vi "Init.vi"(6 "dT (Auto)":dbl, 7 "Output Range":T1={"Min"=-50.0, "Max"=50.0}, 8 "error in (no error)":errorcluster, 11 "Parameters":T2={"P Band"=10.0, "I Gain"=0.5, "D Gain"=0.1, "F Gain"=0.0}) -> (0 "error out":errorcluster, 3 "PID out":refnum<class "PID.lvclass">)   [LabVIEW 2020, in "IG PID.lvlib" / "PID.lvclass"]
uses:
  PID.lvclass
  Parameters.ctl
  Output Range.ctl
  State.ctl
  PID.lvclass/PID.ctl
  IG PID.lvlib
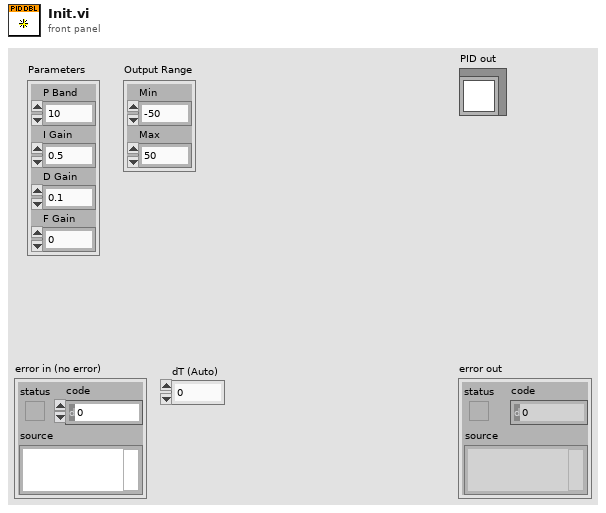
[diagram p1: front panel]
types:
  T1 = typedef "IG PID.lvlib/Output Range.ctl" = cluster{"Min":dbl, "Max":dbl}
  T2 = typedef "IG PID.lvlib/Parameters.ctl" = cluster{"P Band":dbl, "I Gain":dbl, "D Gain":dbl, "F Gain":dbl}
  T3 = typedef "IG PID.lvlib/State.ctl" = cluster{"F":dbl, "P":dbl, "I":dbl, "D":dbl, "Error":dbl, "Sum":dbl, "PV":dbl, "Out":dbl, "dT":dbl, "SP":dbl}
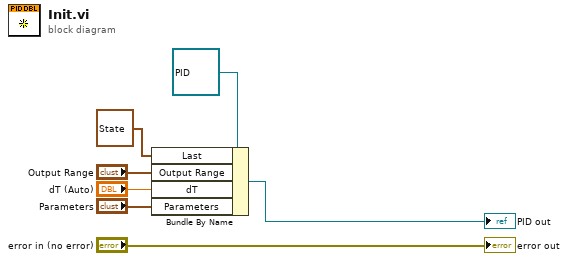
[diagram p0: block diagram]
diagram:
  n1 = Bundle By Name(cluster=refnum<class "PID.lvclass"> refnum ("PID in"), "Last"=T3 {"F"=0.0, "P"=0.0, "I"=0.0, "D"=0.0, "Error"=0.0, "Sum"=0.0, "PV"=0.0, "Out"=0.0, "dT"=0.0, "SP"=0.0}, "Output Range"="Output Range", "dT"="dT (Auto)", "Parameters"="Parameters") -> (→"PID out":refnum<class "PID.lvclass">)
  "error out" <- "error in (no error)"
